vi "Read Async Methods Running.vi"(8 "error in (no error)":errorcluster, 11 "Async Methods Actor in":refnum<class "Async Methods Actor.lvclass">) -> (0 "error out":errorcluster, 2 "Async Methods Running":refnum<notifier>, 3 "Async Methods Actor out":refnum<class "Async Methods Actor.lvclass">)   [LabVIEW 2021, in "Async Methods Actor.lvlib" / "Async Methods Actor.lvclass"]
doc: "The execution of \"Call and Collect\" methods and the launch of \"Call and Forget\" can be followed by subscribing the notifier available from this property."
uses:
  Async Methods Actor.lvclass
  Async Methods Running.ctl
  Async Methods Actor.lvclass/Async Methods Actor.ctl
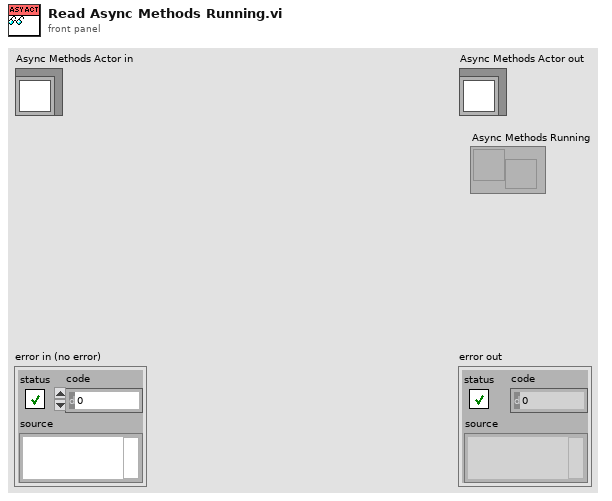
[diagram p1: front panel]
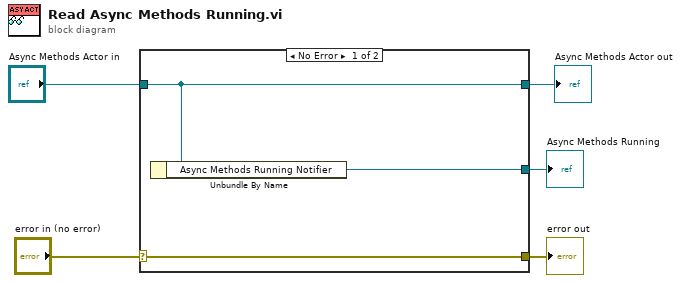
[diagram p0: block diagram]
diagram:
  n1 = case shown="No Error" "error in (no error)" {
    selector: "error in (no error)" -> [w8 w9]
    tunnel: [w8 w9] -> w4
    tunnel: [w7 w10] -> w1
    tunnel: "Async Methods Actor in" -> [w7 w10]
    tunnel: [w6 _] -> w3
    frame No Error {
      n2 = Unbundle By Name(w7) -> ("Async Methods Running Notifier"=w6:refnum<notifier>)
    }
    frame Error {
    }
  }
  "error out" <- w4
  "Async Methods Running" <- w3
  "Async Methods Actor out" <- w1
